vi "Initialize.vi"(8 "error in":errorcluster, 10 "Name":string, 11 "Attribute in":refnum<class "Attribute.lvclass">) -> (0 "error out":errorcluster, 3 "Attribute out":refnum<class "Attribute.lvclass">)   [LabVIEW 2021, in "ProligentXMLGenerator.lvlib" / "Attribute.lvclass"]
uses:
  Attribute.lvclass
  Attribute.lvclass/Attribute.ctl
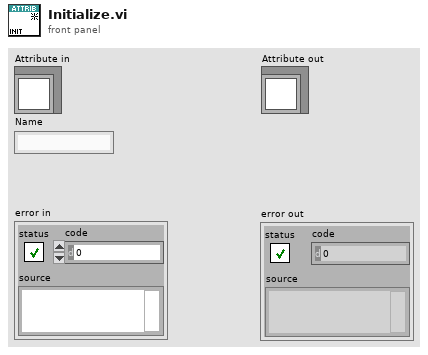
[diagram p1: front panel]
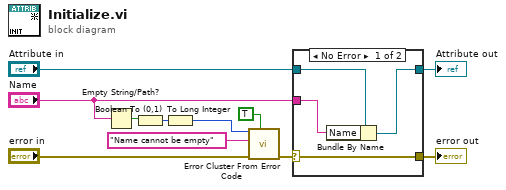
[diagram p0: block diagram]
diagram:
  n1 = Empty String/Path?(string/path="Name") -> (empty?=w9:bool)
  n2 = Boolean To (0,1)(Boolean=w9) -> (0, 1=w8:i16)
  n3 = To Long Integer(number=w8) -> (32bit integer=w7:i32)
  n4 = call <vilib>:"Error Cluster From Error Code.vi"("show call chain? (False)"=TRUE, "error in (no error)"="error in", "error message (\"\")"="Name cannot be empty" ("error message (\"\")"), "error code (0)"=w7) -> ("error out"=w1:errorcluster)  [unwired: 5 in]
  n5 = case shown="No Error" w1 {
    selector: w1 -> [w12 w16]
    tunnel: [w15 w17] -> w5
    tunnel: "Attribute in" -> [w14 w17]
    tunnel: "Name" -> [w13 _]
    tunnel: [w12 w16] -> w2
    frame No Error {
      n6 = Bundle By Name(cluster=w14, "Name"=w13) -> (w15:refnum<class "Attribute.lvclass">)
    }
    frame Error {
    }
  }
  "Attribute out" <- w5
  "error out" <- w2
